vi "StartThread.vi"(0 "reference in":refnum<class "SuperNS.lvclass">, 2 "OpenThreadWin":bool, 5 "error in":errorcluster) -> (14 "reference out":refnum<class "SuperNS.lvclass">, 19 "error out":errorcluster)   [LabVIEW 2018, in "SuperNS.lvclass"]
doc: "Copyright © 2008 - 2024 VI Technologies B.V. \nALL RIGHTS RESERVED"
uses:
  SuperNS.lvclass
  <vilib>/Utility/error.llb/Error Cluster From Error Code.vi
  <vilib>/ErrorRing/Error Ring.xnode
panel:
  # "Copyright (c) 2024, VI Technologies B.V.\nAll rights reserved.\n\nRedistribution and use in source and binary forms, with or without modification, are permitted provided that \nthe following conditions are met:\n\n * Redistributions of source code must retain the above copyright notice, this list of conditions and the \nfollowing disclaimer.\n * Redistributions in binary form must reproduce the above copyright notice, this list of conditions and the \nfollowing disclaimer in the documentation and/or other materials provided with the distribution.\n * Neither the name of VI Technologies B.V. nor the names of its contributors may be used to endorse or \npromote products derived from this software without specific prior written permission.\n\nTHIS SOFTWARE IS PROVIDED BY THE COPYRIGHT HOLDERS AND CONTRIBUTORS \"AS IS\" AND ANY EXPRESS OR \nIMPLIED WARRANTIES, INCLUDING, BUT NOT LIMITED TO, THE IMPLIED WARRANTIES OF MERCHANTABILITY \nAND FITNESS FOR A PARTICULAR PURPOSE ARE DISCLAIMED. IN NO EVENT SHALL THE COPYRIGHT OWNER OR \nCONTRIBUTORS BE LIABLE FOR ANY DIRECT, INDIRECT, INCIDENTAL, SPECIAL, EXEMPLARY, OR CONSEQUENTIAL \nDAMAGES (INCLUDING, BUT NOT LIMITED TO, PROCUREMENT OF SUBSTITUTE GOODS OR SERVICES; LOSS OF \nUSE, DATA, OR PROFITS; OR BUSINESS INTERRUPTION) HOWEVER CAUSED AND ON ANY THEORY OF LIABILITY, \nWHETHER IN CONTRACT, STRICT LIABILITY, OR TORT (INCLUDING NEGLIGENCE OR OTHERWISE) ARISING IN ANY \nWAY OUT OF THE USE OF THIS SOFTWARE, EVEN IF ADVISED OF THE POSSIBILITY OF SUCH DAMAGE.\n\nFor more information, please visit https://www.vi-tech.nl or contact us at info@vi-tech.nl"
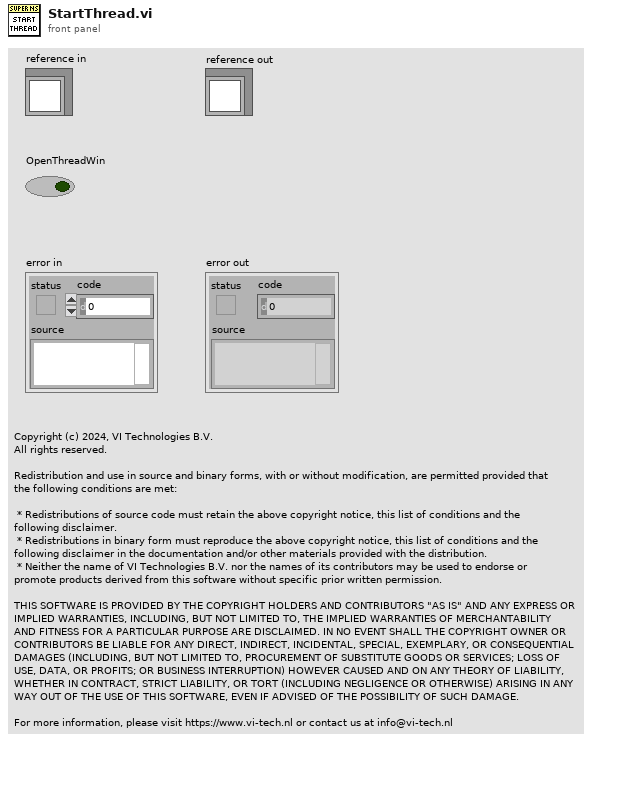
[diagram p1: front panel]
types:
  T1 = typedef "SuperNS.lvclass/ObjectAttributes.ctl" = cluster{"NSName":string, "RemoteEP_URL":string, "BufferSize":i32, "Element Allocation Mode":T2, "ConnLost Timeout":i32, "Writer":bool, "ReadDataEvent":string, "FlushAfterWrite":bool, "Thread":cluster{"VI Refnum":refnum<vi>, "Started Notifier":refnum<notifier>, "Stopped Notifier":refnum<notifier>, "CmdEvent":refnum<user-event>}, "Endpoint":refnum<k21>, "R/W Error":bool, "Flush Wait Condition":T3, "DataReadEvent":refnum<user-event>, "NS Created":bool, "BG ConnCheck/Read period":i32, "ErrorHandler":refnum<class "ErrorHandler.lvclass">}
  T2 = typedef "Stream Element Allocation Mode.ctl" = u32
  T3 = typedef "Flush And Wait Empty Condition.ctl" = u8
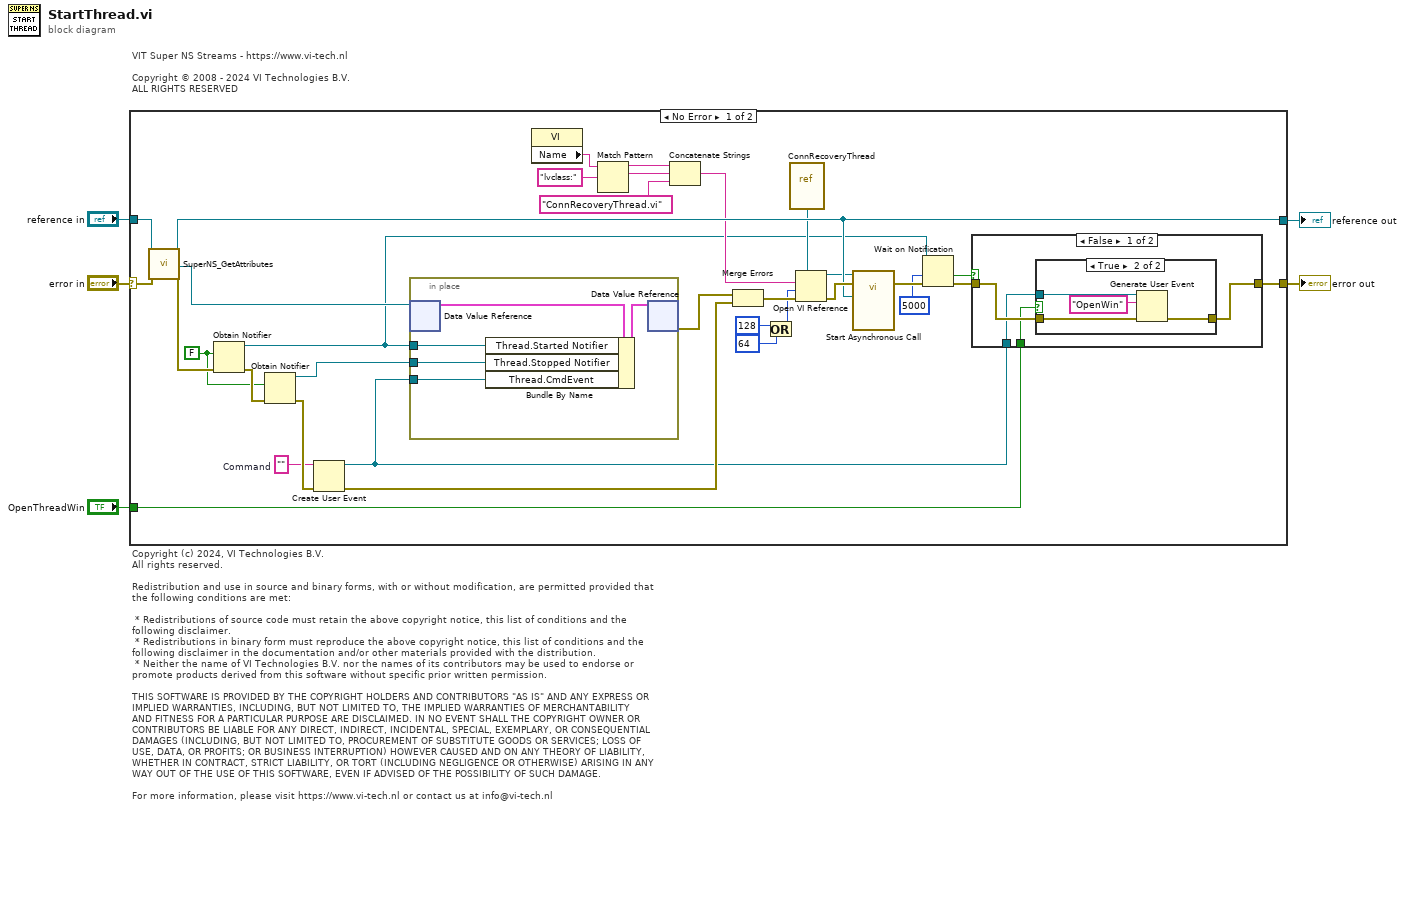
[diagram p0: block diagram]
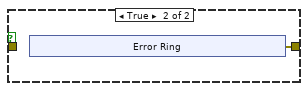
[diagram p3: hidden frame]
diagram:
  # "VIT Super NS Streams - https://www.vi-tech.nl\n\nCopyright © 2008 - 2024 VI Technologies B.V. \nALL RIGHTS RESERVED"
  # "Copyright (c) 2024, VI Technologies B.V.\nAll rights reserved.\n\nRedistribution and use in source and binary forms, with or without modification, are permitted provided that \nthe following conditions are met:\n\n * Redistributions of source code must retain the above copyright notice, this list of conditions and the \nfollowing disclaimer.\n * Redistributions in binary form must reproduce the above copyright notice, this list of conditions and the \nfollowing disclaimer in the documentation and/or other materials provided with the distribution.\n * Neither the name of VI Technologies B.V. nor the names of its contributors may be used to endorse or \npromote products derived from this software without specific prior written permission.\n\nTHIS SOFTWARE IS PROVIDED BY THE COPYRIGHT HOLDERS AND CONTRIBUTORS \"AS IS\" AND ANY EXPRESS OR \nIMPLIED WARRANTIES, INCLUDING, BUT NOT LIMITED TO, THE IMPLIED WARRANTIES OF MERCHANTABILITY \nAND FITNESS FOR A PARTICULAR PURPOSE ARE DISCLAIMED. IN NO EVENT SHALL THE COPYRIGHT OWNER OR \nCONTRIBUTORS BE LIABLE FOR ANY DIRECT, INDIRECT, INCIDENTAL, SPECIAL, EXEMPLARY, OR CONSEQUENTIAL \nDAMAGES (INCLUDING, BUT NOT LIMITED TO, PROCUREMENT OF SUBSTITUTE GOODS OR SERVICES; LOSS OF \nUSE, DATA, OR PROFITS; OR BUSINESS INTERRUPTION) HOWEVER CAUSED AND ON ANY THEORY OF LIABILITY, \nWHETHER IN CONTRACT, STRICT LIABILITY, OR TORT (INCLUDING NEGLIGENCE OR OTHERWISE) ARISING IN ANY \nWAY OUT OF THE USE OF THIS SOFTWARE, EVEN IF ADVISED OF THE POSSIBILITY OF SUCH DAMAGE.\n\nFor more information, please visit https://www.vi-tech.nl or contact us at info@vi-tech.nl"
  n1 = case shown="No Error" "error in" {
    selector: "error in" -> [w38 w60]
    tunnel: [w30 w60] -> w4
    tunnel: [w22 w59] -> w2
    tunnel: "reference in" -> [w27 w59]
    tunnel: "OpenThreadWin" -> [w16 _]
    frame No Error {
      w19 = ""  # Command
      w26 = FALSE
      n2 = call "SuperNS_GetAttributes.vi"("reference in"=w27, "error in"=w38) -> ("reference out"=w22:refnum<class "SuperNS.lvclass">, "DataRef"=w9:refnum<data-value>, "error out"=w37:errorcluster)  [unwired: 14 in, 1 out]
      n3 = Obtain Notifier(notification data type=w26, error in (no error)=w37) -> (notifier out=w8:refnum<notifier>, error out=w36:errorcluster)  [unwired: 2 in, 1 out]
      n4 = Obtain Notifier(notification data type=w26, error in (no error)=w36) -> (notifier out=w7:refnum<notifier>, error out=w35:errorcluster)  [unwired: 2 in, 1 out]
      n5 = Create User Event(user event datatype=w19, error in=w35) -> (user event=w6:refnum<user-event>, error out=w34:errorcluster)
      n6 = in-place {
        in-place-border: w8 -> [w42]
        in-place-border: w7 -> [w41]
        in-place-border: w6 -> [w40]
        n7 = in-place-dvr #1(w9) -> (w39:T1)  [unwired: 1 out]
        n8 = Bundle By Name(cluster=w39, "Thread.Started Notifier"=w42, "Thread.Stopped Notifier"=w41, "Thread.CmdEvent"=w40) -> (w43:T1)
        n9 = in-place-dvr #1(w43) -> (w28:errorcluster)  [unwired: 1 out]
      }
      n10 = property class="VI"() -> ("Name"=w15:string)  [unwired: 2 in, 2 out]
      n11 = Match Pattern(string=w15, regular expression="lvclass:") -> (before substring=w13:string, match substring=w12:string)  [unwired: 1 in, 2 out]
      n12 = Concatenate Strings(w13, w12, "ConnRecoveryThread.vi") -> (w11:string)
      n13 = Merge Errors(w28, w34) -> (w33:errorcluster)
      n14 = Or(x=128 ("options"), y=64) -> (x .or. y?=w24:i32)
      n15 = vi-ref "ConnRecoveryThread.vi"() -> (w18:refnum<vi>)
      n16 = Open VI Reference(type specifier VI Refnum (for type only)=w18, vi path=w11, options=w24, error in (no error)=w33) -> (vi reference=w17:refnum<vi>, error out=w32:errorcluster)  [unwired: 2 in]
      n17 = call-by-ref "Start Asynchronous Call"(reference=w17, error in=w32, "reference in"=w22) -> (error out=w31:errorcluster)  [unwired: 19 in, 1 out]
      n18 = Wait on Notification(notifier=w8, timeout in ms (-1)=5000, error in (no error)=w31) -> (timed out?=w20:bool, error out=w29:errorcluster)  [unwired: 1 in, 2 out]
      n19 = case shown="False" w20 {
        tunnel: [w46 w53] -> w30
        tunnel: w29 -> [w47 _]
        tunnel: w6 -> [w45 _]
        tunnel: w16 -> [w44 _]
        frame False {
          n20 = case shown="True" w44 {
            tunnel: w47 -> [w48 w52]
            tunnel: [w48 w51] -> w46
            tunnel: w45 -> [_ w50]
            frame False {
            }
            frame True {
              n21 = Generate User Event(user event=w50, event data cluster="OpenWin" ("event data"), error in=w52) -> (error out=w51:errorcluster)  [unwired: 1 in, 1 out]
            }
          }
        }
        frame True {
          n22 = xnode "Error Ring"() -> ("error out"=w53:errorcluster)
        }
      }
    }
    frame Error {
    }
  }
  "error out" <- w4
  "reference out" <- w2
